vi "Tree_Open Item and parents.vi"(6 "Close all first [T]":bool=TRUE, 8 "error in (no error)":errorcluster, 10 "Tag":string, 11 "TreeControl in":refnum<vi>) -> (0 "error out":errorcluster)   [LabVIEW 2023]
doc: "Takes a tag (or part of a tag) and opens it and all its parent items"
panel:
  in  "Debug Tree":string[](tree)
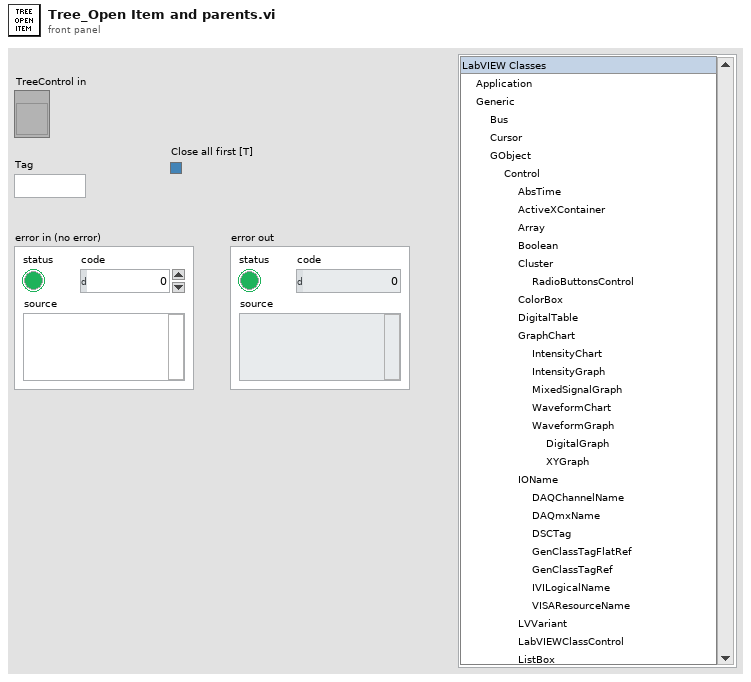
[diagram p1: front panel]
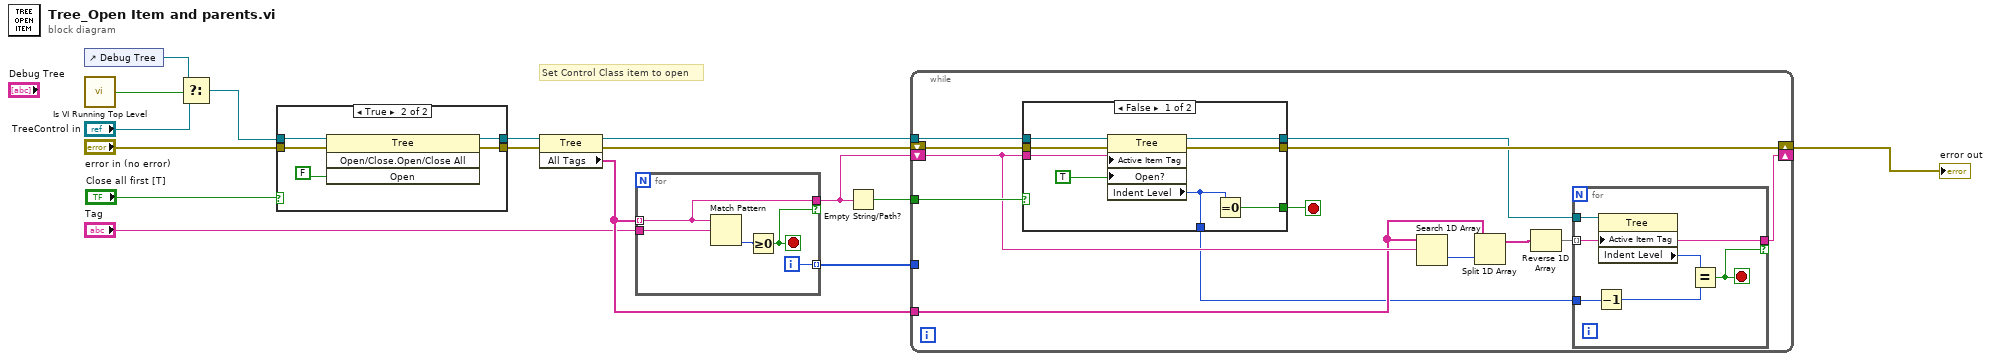
[diagram p0: block diagram]
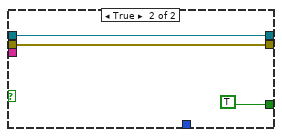
[diagram p3: hidden frame]
diagram:
  # "Set Control Class item to open"
  n1 = control-ref of="Debug Tree"() -> (w5:refnum<vi>)
  n2 = call "Is VI Running Top Level.vi"() -> ("Top Level?"=w8:bool)  [unwired: 5 in]
  n3 = Select(t=w5, s=w8, f="TreeControl in") -> (s? t:f=w6:refnum<vi>)
  n4 = case shown="True" "Close all first [T]" {
    tunnel: w6 -> [w18 w23]
    tunnel: [w18 w22] -> w4
    tunnel: "error in (no error)" -> [w17 w21]
    tunnel: [w17 w20] -> w2
    frame False {
    }
    frame True {
      n5 = invoke class="Tree" method="Open/Close.Open/Close All"(reference=w23, error in=w21, "Open"=FALSE ("Open?")) -> (reference out=w22:refnum<vi>, error out=w20:errorcluster)  [unwired: 1 in, 2 out]
    }
  }
  n6 = property class="Tree"(reference=w4, error in=w2) -> (reference out=w12:refnum<vi>, error out=w15:errorcluster, "All Tags"=w10:string[])
  n7 = for {
    tunnel: w10 -> [w27] mode=indexing
    tunnel: [w27] -> w13 if=w26
    tunnel: [w25] -> w11 mode=indexing
    tunnel: "Tag" -> [w24]
    i -> [w25]
    stop <- w26 stop-if-true
    n8 = Match Pattern(string=w27, regular expression=w24) -> (offset past match=w28:i32)  [unwired: 1 in, 3 out]
    n9 = Greater Or Equal To 0?(x=w28) -> (x >= 0?=w26:bool)
  }
  n10 = Empty String/Path?(string/path=w13) -> (empty?=w14:bool)
  n11 = while {
    tunnel: w14 -> [w39]
    tunnel: w12 -> [w38]
    shift-right: [w41] -> w16
    shift-left: w15 -> [w40]
    tunnel: w11 -> [_]
    tunnel: w10 -> [w34]
    shift-right: [w30] -> _
    shift-left: w13 -> [w36]
    stop <- w37 stop-if-true
    n12 = case shown="False" w39 {
      tunnel: w38 -> [w55 w56]
      tunnel: w36 -> [w54 _]
      tunnel: w40 -> [w52 w58]
      tunnel: [w51 w58] -> w41
      tunnel: [w50 TRUE] -> w37
      tunnel: [w49 _] -> w31
      tunnel: [w48 w56] -> w29
      frame False {
        n13 = property class="Tree"(reference=w55, error in=w52, "Active Item Tag"=w54, "Open?"=TRUE ("Active Item:Open?")) -> (reference out=w48:refnum<vi>, error out=w51:errorcluster, "Indent Level"=w49:i32)
        n14 = Equal To 0?(x=w49) -> (x = 0?=w50:bool)
      }
      frame True {
      }
    }
    n15 = Search 1D Array(1D array=w34, element=w36) -> (index of element=w35:i32)  [unwired: 1 in]
    n16 = Split 1D Array(array=w34, index=w35) -> (first subarray=w33:string[])  [unwired: 1 out]
    n17 = Reverse 1D Array(array=w33) -> (reversed array=w32:string[])
    n18 = for {
      tunnel: w32 -> [w44] mode=indexing
      tunnel: w31 -> [w46]
      tunnel: [w44] -> w30 if=w43
      tunnel: w29 -> [w42]
      stop <- w43 stop-if-true
      n19 = Decrement(x=w46) -> (x-1=w45:i32)
      n20 = property class="Tree"(reference=w42, "Active Item Tag"=w44) -> ("Indent Level"=w47:i32)  [unwired: 1 in, 2 out]
      n21 = Equal?(x=w47, y=w45) -> (x = y?=w43:bool)
    }
  }
  "error out" <- w16
